vi "ExposeGetEventStream.vi"(8 "error in":errorcluster, 10 "Category":string, 11 "ID":string) -> (0 "error out":errorcluster, 1 "Event Stream Info":T3, 2 "EventStream":T2, 3 "Event Registration Refnum out":T1)   [LabVIEW 2017]
uses:
  ExposeEventStreamType.ctl
  ExposeEventStreamDataType.ctl
  ExposeEventType.ctl
  ExposeEventRegistrationDataType.ctl
  ExposeEventGlobals.vi
panel:
  out "Stream Name":string
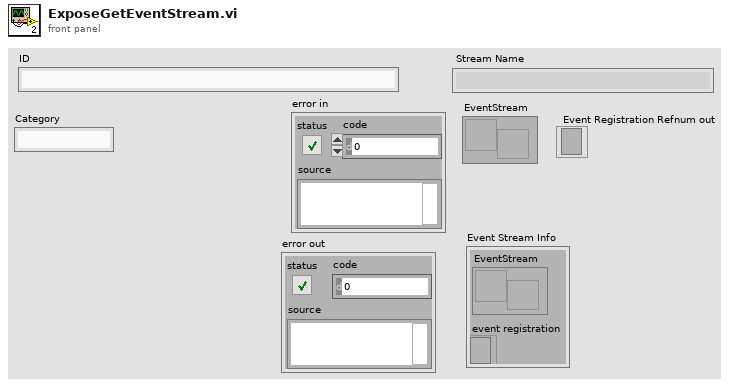
[diagram p1: front panel]
types:
  T1 = typedef "ExposeEventRegistrationDataType.ctl" = refnum<event-registration>
  T2 = typedef "ExposeEventStreamDataType.ctl" = refnum<user-event>
  T3 = typedef "ExposeEventStreamType.ctl" = cluster{"EventStream":T2, "event registration":T1}
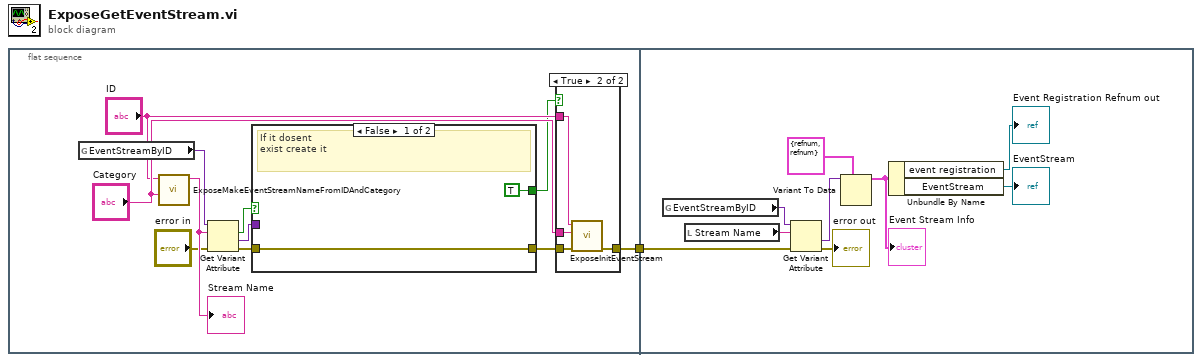
[diagram p0: block diagram]
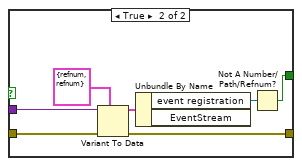
[diagram p3: hidden frame]
diagram:
  n1 = flat-sequence {
    tunnel: [w4] -> w1
    tunnel: w1 -> [w35]
    frame #0 {
      n2 = global read "ExposeEventGlobals.vi" "EventStreamByID"() -> (w8:variant)
      n3 = call "ExposeMakeEventStreamNameFromIDAndCategory.vi"("Category"="Category", "ID"="ID") -> ("StreamName"=w12:string)  [unwired: 9 in]
      "Stream Name" <- w12
      n4 = Get Variant Attribute(Variant=w8, name=w12, error in="error in") -> (found=w11:bool, value=w5:variant, error out=w7:errorcluster)  [unwired: 1 in, 1 out]
      n5 = case shown="False" w11 {
        tunnel: w7 -> [w18 w21]
        tunnel: [w18 w20] -> w2
        tunnel: w5 -> [_ w26]
        tunnel: [TRUE w22] -> w3
        frame False {
          # "If it dosent\nexist create it"
        }
        frame True {
          n6 = Variant To Data(error in=w21, type=T3 {"EventStream"=refnum, "event registration"=refnum} ("EventStreamInfo"), Variant=w26) -> (data=w24:T3, error out=w20:errorcluster)
          n7 = Unbundle By Name(w24) -> ("event registration"=w23:T1)  [unwired: 1 out]
          n8 = Not A Number/Path/Refnum?(number/path/refnum=w23) -> (NaN/Path/Refnum?=w22:bool)
        }
      }
      n9 = case shown="True" w3 {
        tunnel: "Category" -> [_ w17]
        tunnel: "ID" -> [_ w16]
        tunnel: w2 -> [w13 w15]
        tunnel: [w13 w14] -> w4
        frame False {
        }
        frame True {
          n10 = call "ExposeInitEventStream.vi"("error in"=w15, "Category"=w17, "ID"=w16) -> ("error out"=w14:errorcluster)  [unwired: 7 in, 1 out]
        }
      }
    }
    frame #1 {
      n11 = global read "ExposeEventGlobals.vi" "EventStreamByID"() -> (w33:variant)
      n12 = local read "Stream Name"() -> (w27:string)
      n13 = Get Variant Attribute(Variant=w33, name=w27, error in=w35) -> (value=w29:variant, error out=→"error out":errorcluster)  [unwired: 1 in, 2 out]
      n14 = Variant To Data(type=T3 {"EventStream"=refnum, "event registration"=refnum} ("EventStreamInfo"), Variant=w29) -> (data=w32:T3)  [unwired: 1 in, 1 out]
      "Event Stream Info" <- w32
      n15 = Unbundle By Name(w32) -> ("event registration"=→"Event Registration Refnum out":T1, "EventStream"=→"EventStream":T2)
    }
  }
